vi "InitHH_AnyThread.vi"(9 "mode":T2 items=["Histo"=0, "T2"=2, "T3"=3, "Conti"=8], 10 "refsource":T3, 11 "Library Version":string="3.0") -> (0 "error out":errorcluster, 2 "Init Info":T1, 3 "DevIdx":i32)   [LabVIEW 2010]
uses:
  HH_InitInfo.ctl
  HH_MeasMode.ctl
  HH_RefSource.ctl
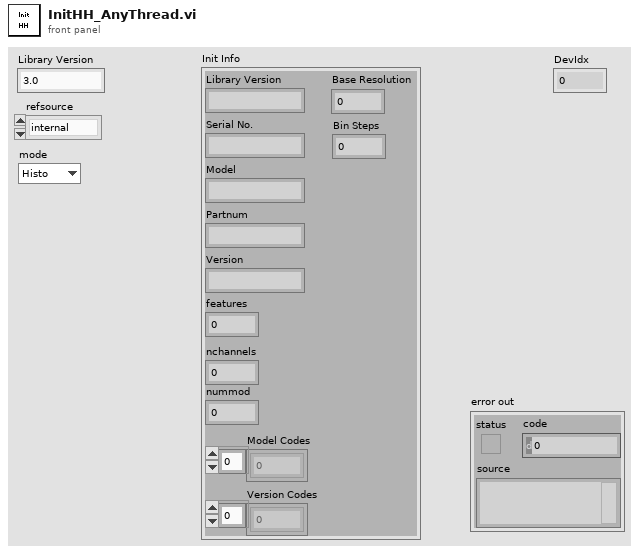
[diagram p1: front panel]
types:
  T1 = typedef "HH_InitInfo.ctl" = cluster{"Library Version":string, "Serial No.":string, "Model":string, "Partnum":string, "Version":string, "features":i32, "nchannels":i32, "nummod":i32, "Model Codes":i32[], "Version Codes":i32[], "Base Resolution":dbl, "Bin Steps":i32}
  T2 = typedef "HH_MeasMode.ctl" = i32
  T3 = typedef "HH_RefSource.ctl" = enum16{"internal", "external"}
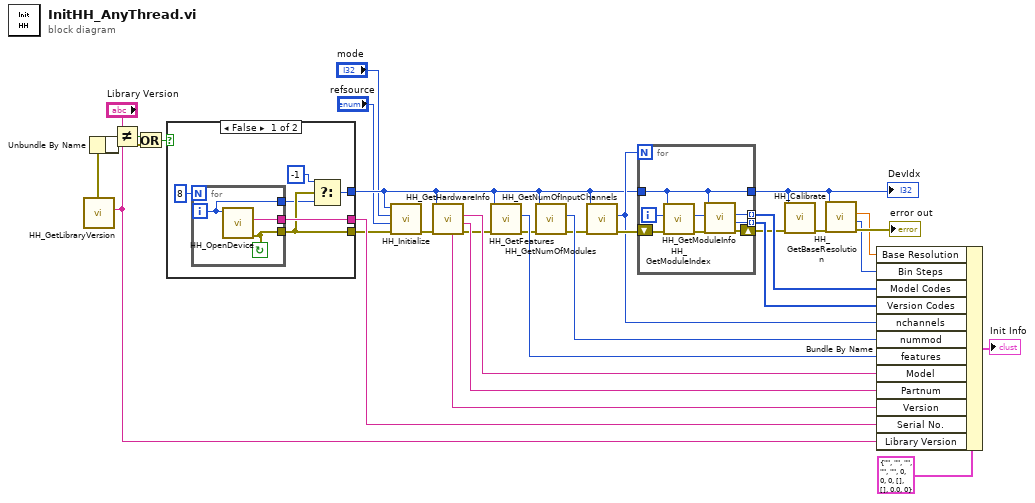
[diagram p0: block diagram]
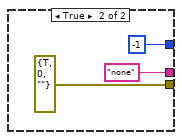
[diagram p2: hidden frame]
diagram:
  n1 = call "HH_GetLibraryVersion.vi"() -> ("error out"=w31:errorcluster, "Version"=w21:string)  [unwired: 9 in, 1 out]
  n2 = Not Equal?(x="Library Version", y=w21) -> (x != y?=w30:bool)
  n3 = Or(x=w30) -> (y=w1:errorcluster, x .or. y?=w29:bool)
  n4 = Unbundle By Name(w31, w1) -> ()
  n5 = case shown="False" w29 {
    tunnel: [w34 -1 ("return type")] -> w5
    tunnel: [w37 "none" ("serial")] -> w23
    tunnel: [w36 errorcluster {"status"=TRUE, "code"=0, "source"=""} ("error out")] -> w2
    frame False {
      n6 = for {
        N: 8 -> [_]
        tunnel: [w40] -> w36
        tunnel: [w39] -> w37
        tunnel: [w41] -> w35
        i -> [w41]
        stop <- w40 continue-if-true
        n7 = call "HH_OpenDevice.vi"("devidx"=w41) -> ("error out"=w40:errorcluster, "serial"=w39:string)  [unwired: 8 in, 1 out]
      }
      n8 = Select(t=-1, s=w36, f=w35) -> (s? t:f=w34:i32)
    }
    frame True {
    }
  }
  n9 = call "HH_Initialize.vi"("error in (no error)"=w2, "refsource"="refsource", "mode"="mode", "devidx"=w5) -> ("error out"=w28:errorcluster)  [unwired: 6 in, 1 out]
  n10 = call "HH_GetHardwareInfo.vi"("error in (no error)"=w28, "devidx"=w5) -> ("error out"=w19:errorcluster, "Partnum"=w26:string, "Model"=w27:string, "Version"=w25:string)  [unwired: 5 in, 1 out]
  n11 = call "HH_GetFeatures.vi"("error in (no error)"=w19, "devidx"=w5) -> ("error out"=w18:errorcluster, "features"=w24:i32)  [unwired: 7 in, 1 out]
  n12 = call "HH_GetNumOfModules.vi"("error in (no error)"=w18, "devidx"=w5) -> ("error out"=w16:errorcluster, "nummod"=w17:i32)  [unwired: 7 in, 1 out]
  n13 = call "HH_GetNumOfInputChannels.vi"("error in (no error)"=w16, "devidx"=w5) -> ("error out"=w15:errorcluster, "nchannels"=w14:i32)  [unwired: 7 in, 1 out]
  n14 = for {
    N: w14 -> [_]
    tunnel: w5 -> [w46]
    tunnel: [w49] -> w13 mode=indexing
    tunnel: [w48] -> w12 mode=indexing
    tunnel: [w46] -> w9
    shift-right: [w45] -> w11
    shift-left: w15 -> [w52]
    i -> [w47]
    n15 = call "HH_GetModuleIndex.vi"("error in (no error)"=w52, "channel"=w47, "devidx"=w46) -> ("error out"=w50:errorcluster, "modidx"=w51:i32)  [unwired: 6 in, 1 out]
    n16 = call "HH_GetModuleInfo.vi"("error in (no error)"=w50, "modidx"=w51, "devidx"=w46) -> ("error out"=w45:errorcluster, "versioncode"=w49:i32, "modelcode"=w48:i32)  [unwired: 5 in, 1 out]
  }
  "DevIdx" <- w9
  n17 = call "HH_Calibrate.vi"("error in (no error)"=w11, "devidx"=w9) -> ("error out"=w10:errorcluster)  [unwired: 8 in, 1 out]
  n18 = call "HH_GetBaseResolution.vi"("error in (no error)"=w10, "devidx"=w9) -> ("error out"=→"error out":errorcluster, "binsteps"=w7:i32, "resolution"=w6:dbl)  [unwired: 6 in, 1 out]
  n19 = Bundle By Name(cluster=T1 {"Library Version"="", "Serial No."="", "Model"="", "Partnum"="", "Version"="", "features"=0, "nchannels"=0, "nummod"=0, "Model Codes"=[], "Version Codes"=[], "Base Resolution"=0.0, "Bin Steps"=0} ("Init"), "Base Resolution"=w6, "Bin Steps"=w7, "Model Codes"=w12, "Version Codes"=w13, "nchannels"=w14, "nummod"=w17, "features"=w24, "Model"=w27, "Partnum"=w26, "Version"=w25, "Serial No."=w23, "Library Version"=w21) -> (→"Init Info":T1)
